vi "Moment Score Coral.vi"(11 "Moment Factor":dbl) -> (3 "Score":dbl)   [LabVIEW 2025]
doc: "Calculate a score based on moment of inertia. There are many forms and this VI uses a normalized form that is more stable and is referred to as Type Factor."
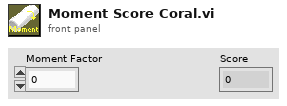
[diagram p1: front panel]
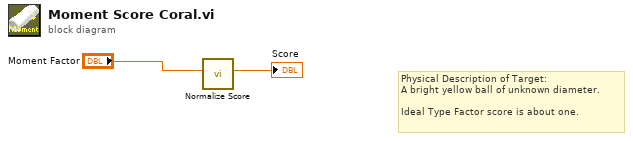
[diagram p0: block diagram]
diagram:
  # "Physical Description of Target:\nA bright yellow ball of unknown diameter.\n\nIdeal Type Factor score is about one."
  n1 = call "Normalize Score.vi"("Value"="Moment Factor") -> ("Score"=→"Score":dbl)  [unwired: 10 in]
